vi "Mode Check.vi"(8 "error in (no error)":errorcluster, 11 "Cfg Grandmaster in":refnum<class "Cfg Grandmaster.lvclass">) -> (0 "error out":errorcluster, 3 "Cfg Grandmaster out":refnum<class "Cfg Grandmaster.lvclass">)   [LabVIEW 2018, in "Configuration Grandmaster.lvlib" / "Cfg Grandmaster.lvclass"]
uses:
  Cfg Grandmaster.lvclass
  Cfg Grandmaster.lvclass/Cfg Grandmaster.ctl
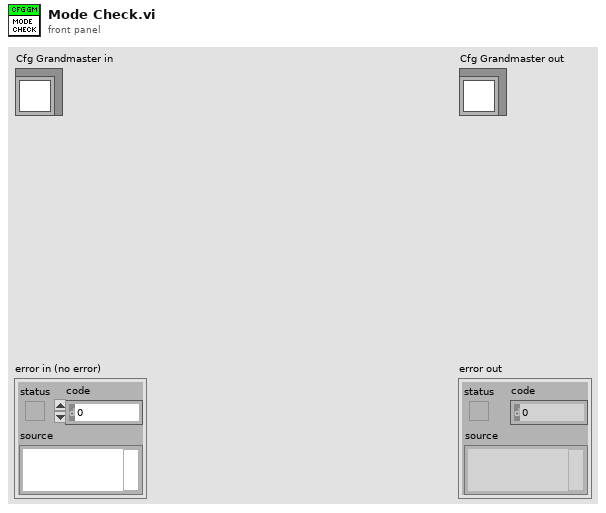
[diagram p1: front panel]
types:
  T1 = typedef "DAQMan Mode.ctl" = enum16{"Cfg", "Run", "Shutting Down"}
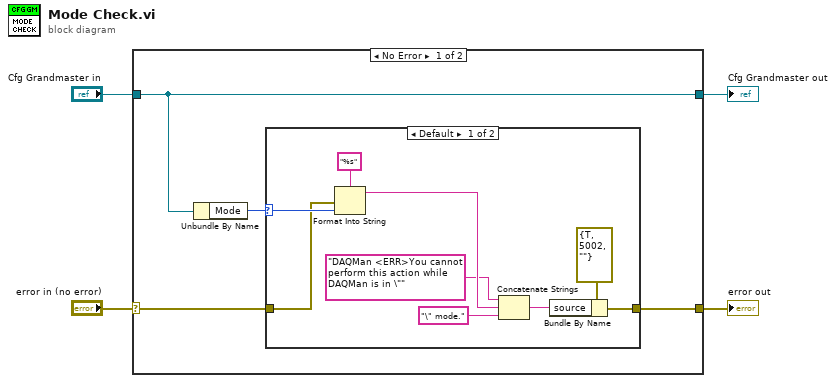
[diagram p0: block diagram]
diagram:
  n1 = case shown="No Error" "error in (no error)" {
    selector: "error in (no error)" -> [w8 w20]
    tunnel: [w7 w20] -> w3
    tunnel: [w6 w19] -> w1
    tunnel: "Cfg Grandmaster in" -> [w6 w19]
    frame No Error {
      n2 = Unbundle By Name(w6) -> ("Mode"=w5:T1)
      n3 = case shown="Default" w5 {
        selector: w5 -> [w11 _]
        tunnel: [w17 w18] -> w7
        tunnel: w8 -> [w10 w18]
        frame Default {
          n4 = Format Into String(format string="%s", error in=w10, w11) -> (resulting string=w14:string)  [unwired: 1 in, 1 out]
          n5 = Concatenate Strings("DAQMan <ERR>You cannot perform this action while DAQMan is in \"", w14, "\" mode." ("string")) -> (w16:string)
          n6 = Bundle By Name(cluster=errorcluster {"status"=TRUE, "code"=5002, "source"=""} ("error out"), "source"=w16) -> (w17:errorcluster)
        }
        frame "Cfg" {
        }
      }
    }
    frame Error {
    }
  }
  "error out" <- w3
  "Cfg Grandmaster out" <- w1
